vi "Set RHS.vi"(8 "error in (no error)":errorcluster, 10 "RHS":variant, 11 "RHS_2D_VIRef in":refnum<class "NI_RHS_2D_VIRef.lvclass">) -> (0 "error out":errorcluster, 3 "RHS_2D_VIRef out":refnum<class "NI_RHS_2D_VIRef.lvclass">)   [LabVIEW 2017, in "NI_PDE.lvlib" / "NI_RHS_2D_VIRef.lvclass"]
uses:
  <vilib>/gmath/pde.llb/RHSClass/RHS_2D_VIRef/NI_RHS_2D_VIRef.lvclass
  <vilib>/gmath/pde.llb/RHSClass/RHS_2D_VIRef/RHS Data.ctl
  <vilib>/gmath/pde.llb/RHSClass/RHS_2D_VIRef/NI_RHS_2D_VIRef.lvclass/NI_RHS_2D_VIRef.ctl
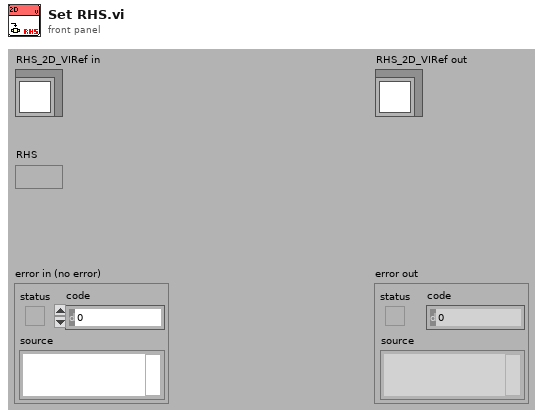
[diagram p1: front panel]
types:
  T1 = typedef "NI_PDE.lvlib/NI_RHS_2D_VIRef.lvclass/RHS Data.ctl" = cluster{"F":refnum<vi>, "data":variant}
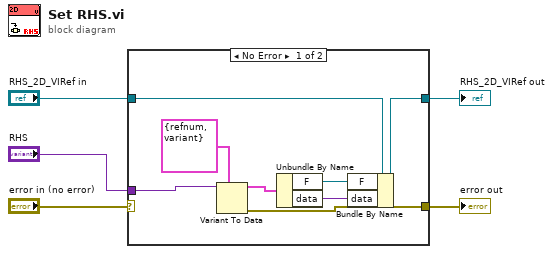
[diagram p0: block diagram]
diagram:
  n1 = case shown="No Error" "error in (no error)" {
    selector: "error in (no error)" -> [_ w15]
    tunnel: "RHS_2D_VIRef in" -> [w10 w14]
    tunnel: [w9 w14] -> w5
    tunnel: [w8 w15] -> w4
    tunnel: "RHS" -> [w13 _]
    frame No Error {
      n2 = Variant To Data(type=T1 {"F"=refnum, "data"=variant} ("RHS data"), Variant=w13) -> (data=w12:T1, error out=w8:errorcluster)  [unwired: 1 in]
      n3 = Unbundle By Name(w12) -> ("F"=w7:refnum<vi>, "data"=w6:variant)
      n4 = Bundle By Name(cluster=w10, "F"=w7, "data"=w6) -> (w9:refnum<class "NI_RHS_2D_VIRef.lvclass">)
    }
    frame Error {
    }
  }
  "RHS_2D_VIRef out" <- w5
  "error out" <- w4
